vi "泵温度校准配置.vi"() -> ()   [LabVIEW 2016, in "斯坦道CODMn新电路板.lvlib"]
uses:
  <vilib>/Utility/miscctls.llb/LVPointTypeDef.ctl
panel:
  in  "关闭":bool
  in  "偏心轮校准簇":T1={"复位"=FALSE, "进水样"=FALSE, "停止"=FALSE, "液体重量"=60, "偏心轮校准"=FALSE}
  in  "温度校准簇":T2={"进水样"=FALSE, "排液"=FALSE, "停止 2"=FALSE, "开始加热"=FALSE, "温度值"=85.0, "温度校准"=FALSE}
  # "偏心轮、温度校准"
  # "输入实际液体重量:"
  # "g"
  # "温度:"
  # "℃"
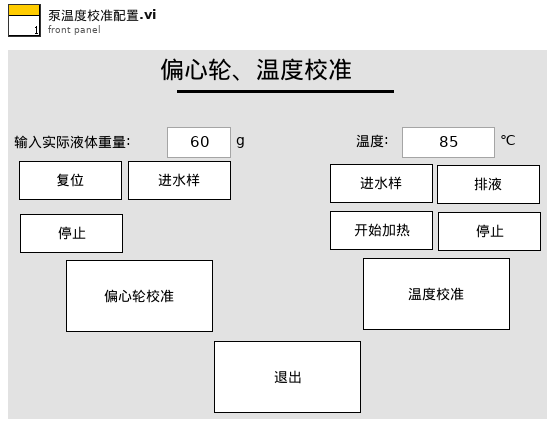
[diagram p1: front panel]
types:
  T1 = cluster{"复位":bool, "进水样":bool, "停止":bool, "液体重量":u16, "偏心轮校准":bool}
  T2 = cluster{"进水样":bool, "排液":bool, "停止 2":bool, "开始加热":bool, "温度值":dbl, "温度校准":bool}
  T3 = typedef "LVPointTypeDef.ctl" = cluster{"Horizontal":i16, "Vertical":i16}
  T4 = cluster{"系统时间":timestamp, "工作状态":u16, "测量模式":enum16{"待机", "连续模式", "周期模式", "定点模式", "受控模式", "手动模式"}, "告警代码":u16, "故障代码":u16, "日志代码":u16, "软件版本":u16, "A":sgl, "B":sgl, "K":sgl, "当前滴定数":sgl, "T":sgl, "H":sgl, "id":u16, "flowid":u16, "量程":u16, "加热实时温度":sgl, "当前ORP值":sgl, "运行时间":sgl, "当前步骤剩余时间":sgl, "结束滴定数":sgl, "注射泵保温温度":sgl}
  T5 = cluster{"偏心轮校准参数":dbl, "运行速度(修改需要重启)":u16, "加热温度(校准参数) ":dbl, "告警温度":dbl, "加热超时时间:(单位/秒)":dbl, "K p":dbl, "K i":dbl, "K d":dbl, "ILimitUp":dbl, "ILimitDown":dbl}
  T6 = cluster{"泵类型":u8, "阀数量":u8, "纯水通道":u8, "废液通道":u8, "进样速度":u16, "出样速度":u16, "滴定速度":u16, "注射泵保温温度L":u8, "注射泵保温温度H":u8, "注射泵加热超时时间":u16, "是否存在液位检测板":u16}
  T7 = cluster{"检出限":dbl, "测量精度":dbl, "上限":dbl, "下限":dbl, "阈值（低->高）":dbl, "阈值（高->低）":dbl}
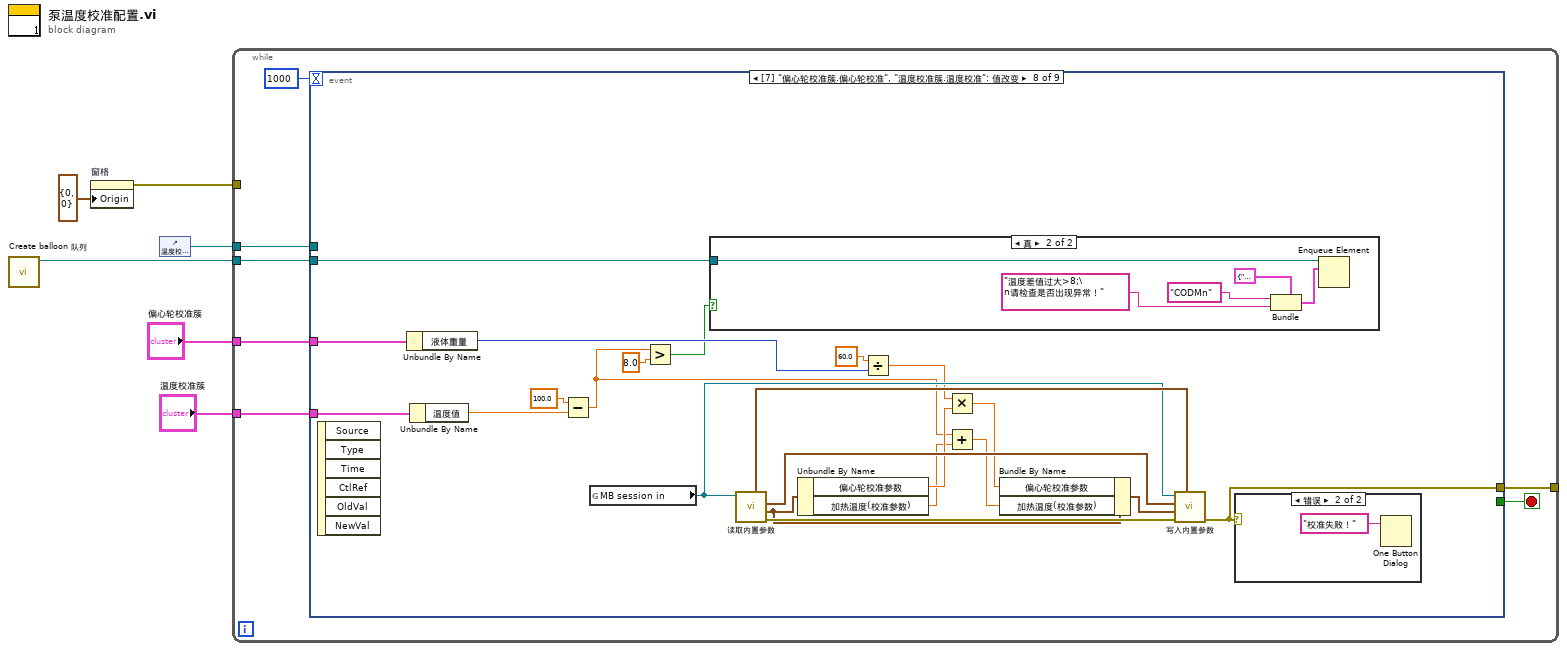
[diagram p0: block diagram]
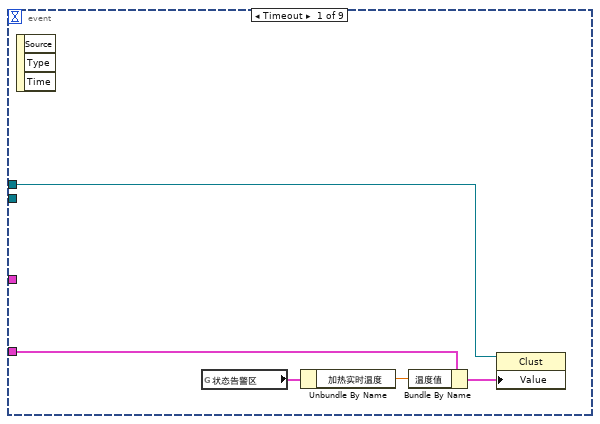
[diagram p2: hidden frame]
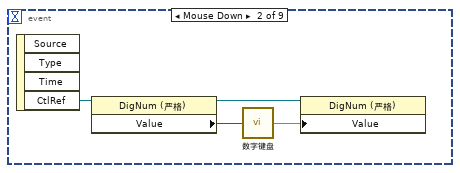
[diagram p3: hidden frame]
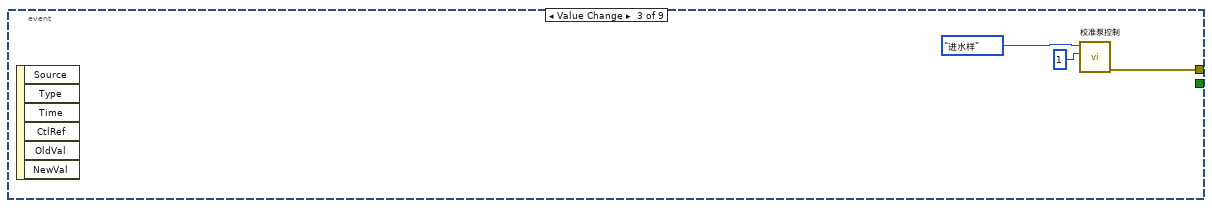
[diagram p4: hidden frame]
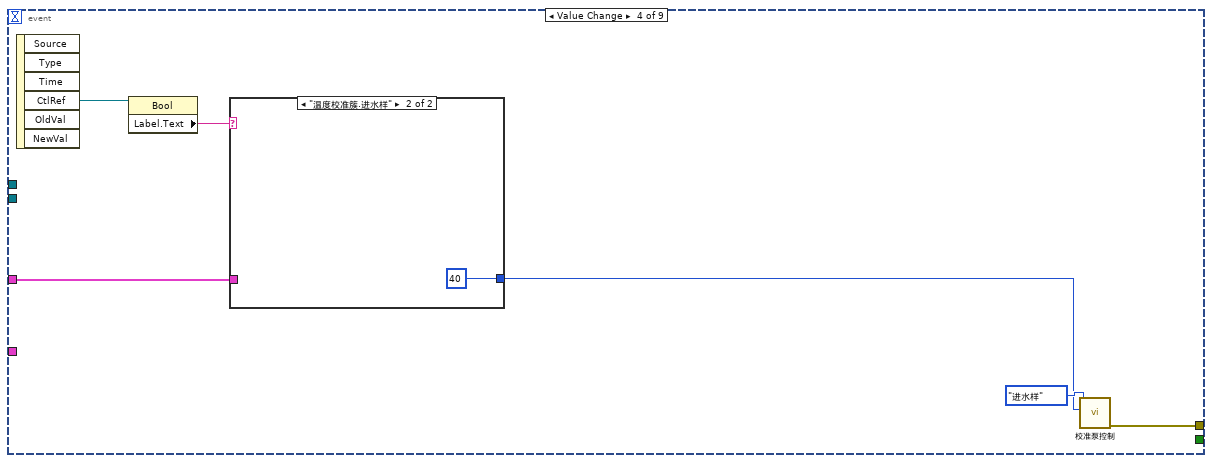
[diagram p5: hidden frame]
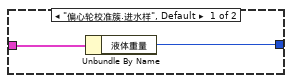
[diagram p6: hidden frame]
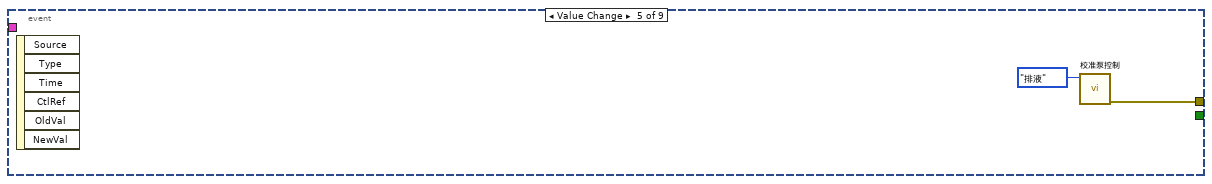
[diagram p7: hidden frame]
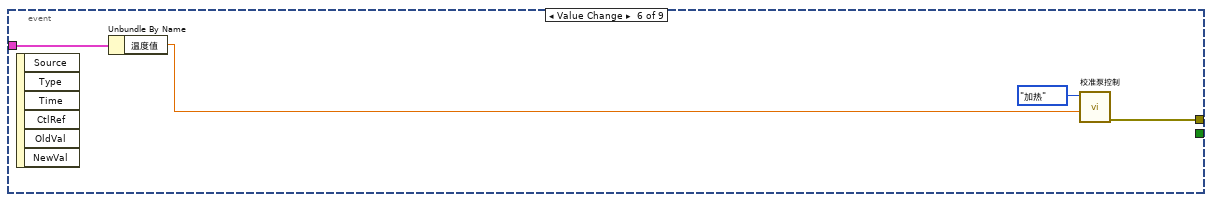
[diagram p8: hidden frame]
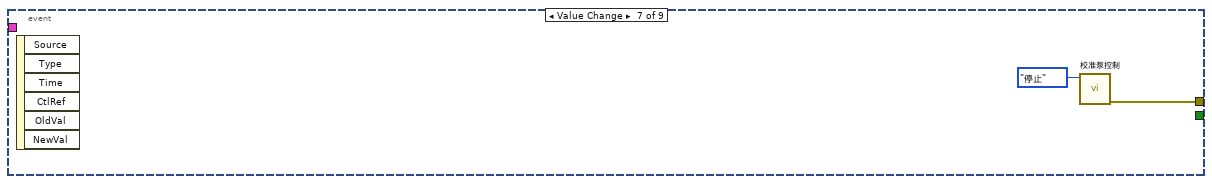
[diagram p9: hidden frame]
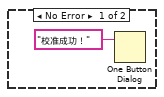
[diagram p11: hidden frame]
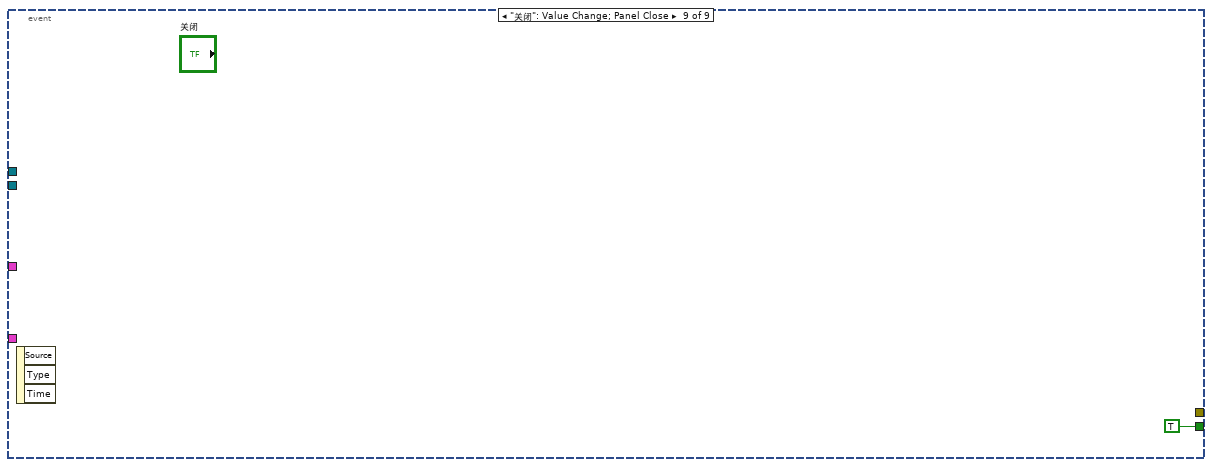
[diagram p12: hidden frame]
diagram:
  n1 = call "Create balloon 队列.vi"() -> ("队列输出"=w1:refnum<queue>)  [unwired: 11 in]
  n2 = property on="窗格" class="Pane"("Origin"=T3 {"Horizontal"=0, "Vertical"=0} ("原点")) -> (error out=w6:errorcluster)  [unwired: 2 in, 1 out]
  n3 = control-ref of="温度校准簇"() -> (w2:refnum<vi>)
  n4 = while {
    tunnel: w6 -> [_]
    tunnel: "偏心轮校准簇" -> [w12]
    tunnel: [w11] -> _
    tunnel: "温度校准簇" -> [w10]
    tunnel: w2 -> [w8]
    tunnel: w1 -> [w7]
    stop <- w13 stop-if-true
    n5 = event shown="[7] \"偏心轮校准簇.偏心轮校准\", \"温度校准簇.温度校准\": 值改变" {
      selector: _ -> [_ _ _ _ _ _ _ _ _]
      dyn-events: _ -> [_ _ _ _ _ _ _ _ _]
      timeout: 1000 -> [_ _ _ _ _ _ _ _ _]
      tunnel: [_ _ _ _ _ _ _ _ TRUE] -> w13
      tunnel: w12 -> [_ _ _ w27 _ _ _ w57 _]
      tunnel: [_ _ w23 w30 w35 w37 w41 w61 _] -> w11
      tunnel: w10 -> [w17 _ _ _ _ w39 _ w55 _]
      tunnel: w8 -> [w15 _ _ _ _ _ _ _ _]
      tunnel: w7 -> [_ _ _ _ _ _ _ w46 _]
      event Timeout {
        n6 = event-data() -> ()  [unwired: 1 in, 3 out]
        n7 = global read "VARCODMn全局变量.vi" "状态告警区"() -> (w18:T4)
        n8 = Unbundle By Name(w18) -> ("加热实时温度"=w16:sgl)
        n9 = Bundle By Name(cluster=w17, "温度值"=w16) -> (w14:T2)
        n10 = property class="Clust"(reference=w15, "Value"=w14) -> ()  [unwired: 1 in, 2 out]
      }
      event "偏心轮校准簇.液体重量": Mouse Down {
        n11 = event-data() -> ("CtlRef"=w19:refnum<vi>)  [unwired: 1 in, 3 out]
        n12 = property class="DigNum (严格)"(reference=w19) -> (reference out=w21:refnum<vi>, "Value"=w22:u16)  [unwired: 1 in, 1 out]
        n13 = call "数字键盘.vi"("OldNumber"=w22) -> ("NewNumber"=w20:dbl)
        n14 = property class="DigNum (严格)"(reference=w21, "Value"=w20) -> ()  [unwired: 1 in, 2 out]
      }
      event "偏心轮校准簇.复位": Value Change {
        n15 = event-data() -> ()  [unwired: 1 in, 6 out]
        n16 = call "校准泵控制.vi"("偏心轮"=u16 1, "枚举"=enum16{"进水样", "排液", "加热", "停止"}."进水样") -> ("错误输出"=w23:errorcluster)  [unwired: 9 in]
      }
      event "偏心轮校准簇.进水样", "温度校准簇.进水样": Value Change {
        n17 = event-data() -> ("CtlRef"=w29:refnum<vi>)  [unwired: 1 in, 5 out]
        n18 = property class="Bool"(reference=w29) -> ("Label.Text"=w28:string)  [unwired: 1 in, 2 out]
        n19 = case shown="\"温度校准簇.进水样\"" w28 {
          tunnel: w27 -> [w33 _]
          tunnel: [w32 u16 40 ("液体重量")] -> w26
          frame "偏心轮校准簇.进水样", Default {
            n20 = Unbundle By Name(w33) -> ("液体重量"=w32:u16)
          }
          frame "温度校准簇.进水样" {
          }
        }
        n21 = call "校准泵控制.vi"("偏心轮"=w26, "枚举"=enum16{"进水样", "排液", "加热", "停止"}."进水样") -> ("错误输出"=w30:errorcluster)  [unwired: 9 in]
      }
      event "温度校准簇.排液": Value Change {
        n22 = event-data() -> ()  [unwired: 1 in, 6 out]
        n23 = call "校准泵控制.vi"("枚举"=enum16{"进水样", "排液", "加热", "停止"}."排液") -> ("错误输出"=w35:errorcluster)  [unwired: 10 in]
      }
      event "温度校准簇.开始加热": Value Change {
        n24 = event-data() -> ()  [unwired: 1 in, 6 out]
        n25 = Unbundle By Name(w39) -> ("温度值"=w38:dbl)
        n26 = call "校准泵控制.vi"("摄氏度"=w38, "枚举"=enum16{"进水样", "排液", "加热", "停止"}."加热") -> ("错误输出"=w37:errorcluster)  [unwired: 9 in]
      }
      event "温度校准簇.停止 2", "偏心轮校准簇.停止": Value Change {
        n27 = event-data() -> ()  [unwired: 1 in, 6 out]
        n28 = call "校准泵控制.vi"("枚举"=enum16{"进水样", "排液", "加热", "停止"}."停止") -> ("错误输出"=w41:errorcluster)  [unwired: 10 in]
      }
      event "偏心轮校准簇.偏心轮校准", "温度校准簇.温度校准": Value Change {
        n29 = event-data() -> ()  [unwired: 1 in, 6 out]
        n30 = Unbundle By Name(w57) -> ("液体重量"=w53:u16)
        n31 = Unbundle By Name(w55) -> ("温度值"=w49:dbl)
        n32 = Subtract(x=100.0, y=w49) -> (x-y=w45:dbl)
        n33 = global read "VARCODMn全局变量.vi" "MB session in"() -> (w62:refnum<class "MB_Master.lvclass">)
        n34 = Greater?(x=w45, y=8.0) -> (0:w43:bool)
        n35 = case shown="真" w43 {
          tunnel: w46 -> [_ w69]
          frame False {
          }
          frame True {
            n36 = Bundle(cluster=cluster{"Title":string, "Body":string} {"Title"="", "Body"=""} ("元素"), "Title"="CODMn", "Body"="温度差值过大>8;\n请检查是否出现异常！") -> (w65:cluster{"Title":string, "Body":string})
            n37 = Enqueue Element(queue=w69, element=w65) -> ()  [unwired: 2 in, 3 out]
          }
        }
        n38 = call "读取内置参数.vi"("MB session in"=w62) -> ("error out"=w64:errorcluster, "float"=w59:T5, "外设配置"=w60:T6, "量程参数读取"=w63:T7)  [unwired: 6 in, 1 out]
        n39 = Unbundle By Name(w59) -> ("偏心轮校准参数"=w52:dbl, "加热温度(校准参数)"=w48:dbl)
        n40 = Divide(x=60.0, y=w53) -> (x/y=w54:dbl)
        n41 = Multiply(x=w54, y=w52) -> (x*y=w51:dbl)
        n42 = Add(x=w45, y=w48) -> (x+y=w47:dbl)
        n43 = Bundle By Name(cluster=w59, "偏心轮校准参数"=w51, "加热温度(校准参数)"=w47) -> (w58:T5)
        n44 = call "写入内置参数.vi"("量程参数读取"=w63, "error in (no error)"=w64, "float"=w58, "外设配置"=w60, "MB session in"=w62) -> ("error out"=w61:errorcluster)  [unwired: 5 in, 1 out]
        n45 = case shown="错误" w61 {
          frame No Error {
            n46 = One Button Dialog(message="校准成功！" ("消息")) -> ()  [unwired: 1 in, 1 out]
          }
          frame Error {
            n47 = One Button Dialog(message="校准失败！" ("消息")) -> ()  [unwired: 1 in, 1 out]
          }
        }
      }
      event "关闭": Value Change; Panel Close {
        n48 = event-data() -> ()  [unwired: 1 in, 3 out]
      }
    }
  }
